vi "unity-connection-test.vi"() -> ()   [LabVIEW 2025]
panel:
  out "Waveform Chart":dbl(graph)
  in  "stop":bool
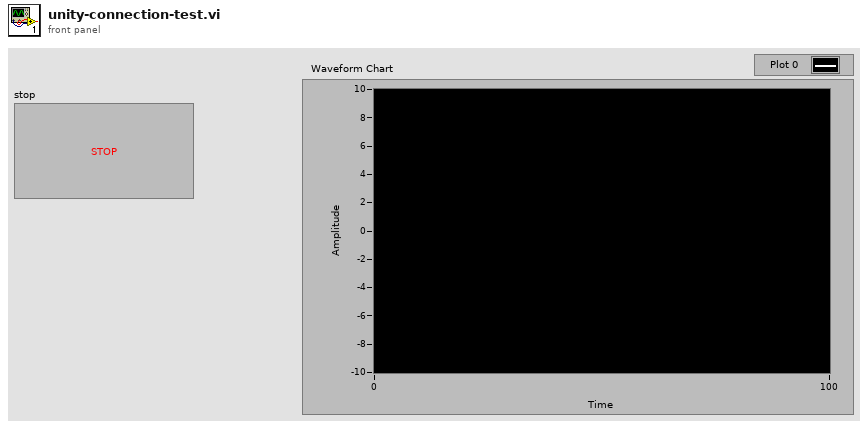
[diagram p1: front panel]
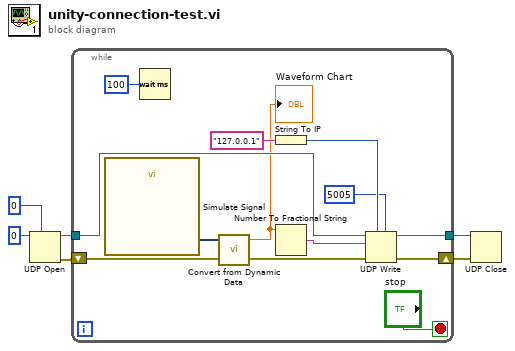
[diagram p0: block diagram]
diagram:
  n1 = UDP Open(7:u32 0 ("net address"), 11:u16 0 ("port")) -> (port=w6:refnum<k16>, 0:w5:errorcluster)  [unwired: 3 in, 1 out]
  n2 = while {
    tunnel: w6 -> [w16]
    tunnel: [w14] -> w4
    shift-right: [w7] -> w1
    shift-left: w5 -> [w15]
    stop <- "stop" stop-if-true
    n3 = call "Simulate Signal"() -> ("Sine"=w17:dynamicdata)  [unwired: 14 in, 1 out]
    n4 = Wait (ms)(milliseconds to wait=u32 100) -> ()  [unwired: 1 out]
    n5 = call "Convert from Dynamic Data"("Dynamic Data Type"=w17) -> ("Scalar"=w8:dbl)  [unwired: 3 in]
    "Waveform Chart" <- w8
    n6 = String To IP(1:"127.0.0.1" ("name")) -> (0:w13:u32)
    n7 = Number To Fractional String(number=w8) -> (F-format string=w10:string)  [unwired: 3 in]
    n8 = UDP Write(address=w13, port or service name=u16 5005, connection ID=w16, data in=w10, 8:w15) -> (error out=w7:errorcluster, 3:w14:refnum<k16>)  [unwired: 1 in]
  }
  n9 = UDP Close(connection ID=w4, 8:w1) -> ()  [unwired: 2 out]
